vi "decodeDataIdentity.vi"(2 "dataIdentityCode":string) -> (3 "VarableID":T1, 4 "dataFormat":string, 5 "unit":string, 6 "dataIdentityText":string)   [LabVIEW 2010]
uses:
  types/VarableID.ctl
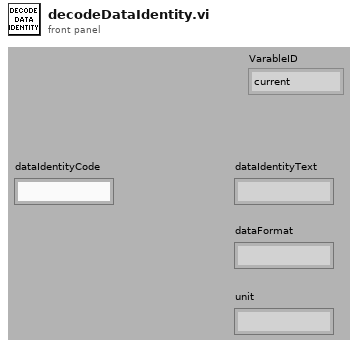
[diagram p1: front panel]
types:
  T1 = typedef "VarableID.ctl" = enum16{"current", "power", "PF", "voltage"}
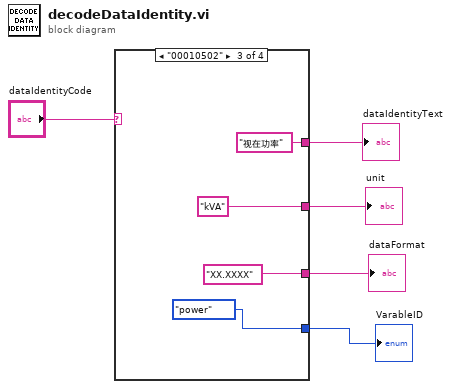
[diagram p0: block diagram]
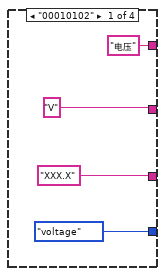
[diagram p2: hidden frame]
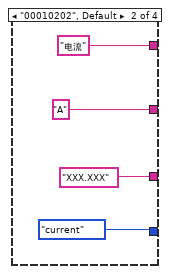
[diagram p3: hidden frame]
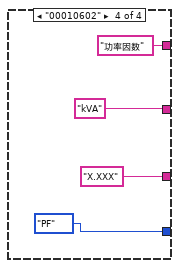
[diagram p4: hidden frame]
diagram:
  n1 = case shown="\"00010502\"" "dataIdentityCode" {
    tunnel: ["电压" "电流" "视在功率" "功率因数"] -> w4
    tunnel: ["V" "A" "kVA" "kVA"] -> w3
    tunnel: ["XXX.X" "XXX.XXX" "XX.XXXX" "X.XXX"] -> w2
    tunnel: [VarableID."voltage" ("VarableID") VarableID."current" ("VarableID") VarableID."power" ("VarableID") VarableID."PF" ("VarableID")] -> w1
    frame "00010102" {
    }
    frame "00010202", Default {
    }
    frame "00010502" {
    }
    frame "00010602" {
    }
  }
  "dataIdentityText" <- w4
  "unit" <- w3
  "dataFormat" <- w2
  "VarableID" <- w1
